vi "ToDegressSetpoint.vi"(4 "Range":cluster{"output high":dbl, "output low":dbl}={"output high"=0.6, "output low"=-0.6} {"output low" format="%.2f"; "output high" format="%.2f"}, 5 "Delay After":i32, 6 "Gains":T1={"proportional gain (Kc)"=1.0, "integral time (Ti, min)"=0.01, "derivative time (Td, min)"=0.0} {"derivative time (Td, min)" format="%.3f"; "integral time (Ti, min)" format="%.3f"; "proportional gain (Kc)" format="%.3f"}, 7 "Loop Wait Delay":i32, 8 "Reset":bool, 9 "Precision":dbl, 10 "Yaw":dbl, 11 "Setpoint (degress)":dbl) -> (0 "Finished?":bool, 3 "Output":dbl)   [LabVIEW 2019]
panel:
  out "PID":cluster{"Distance":dbl, "Encoder Count":dbl}(graph)
  in  "Integral Range":dbl=10000.0
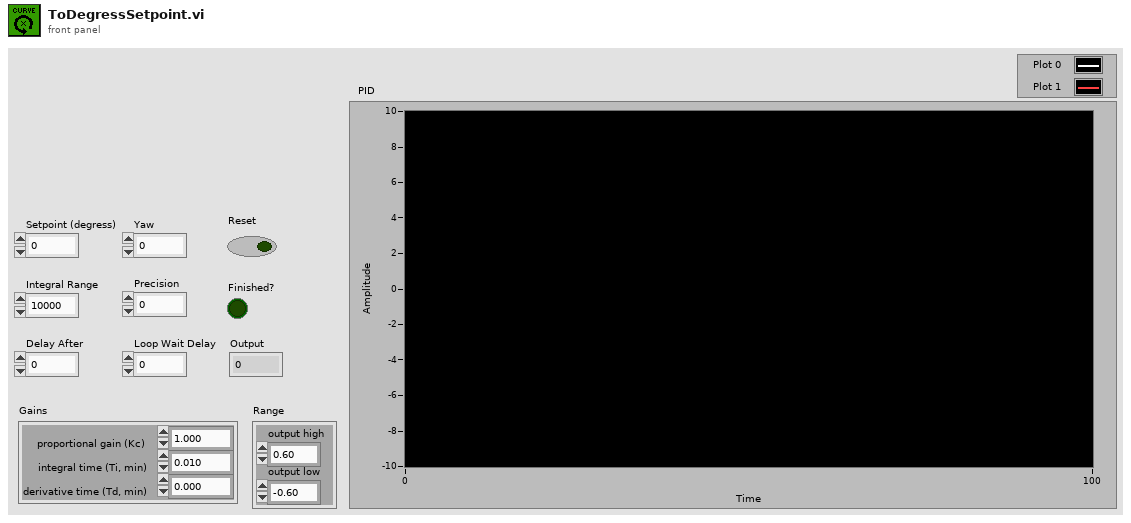
[diagram p1: front panel]
types:
  T1 = cluster{"proportional gain (Kc)":dbl, "integral time (Ti, min)":dbl, "derivative time (Td, min)":dbl}
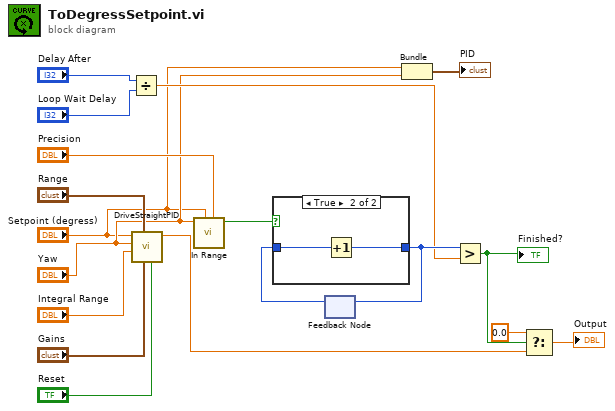
[diagram p0: block diagram]
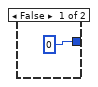
[diagram p2: hidden frame]
diagram:
  n1 = Divide(x="Delay After", y="Loop Wait Delay") -> (x/y=w5:dbl)
  n2 = call "DriveStraightPID.vi"("Reset"="Reset", "Gains"="Gains", "Range"="Range", "Integral Range"="Integral Range", "Process variable"="Yaw", "Setpoint"="Setpoint (degress)") -> ("output"=w8:dbl)  [unwired: 5 in]
  n3 = call "In Range.vi"("Range"="Precision", "Setpoint"="Setpoint (degress)", "Value"="Yaw") -> ("in range?"=w12:bool)  [unwired: 8 in]
  n4 = feedback #1() -> (w10:i32)  [unwired: 1 in]
  n5 = case shown="True" w12 {
    tunnel: [0 w20] -> w6
    tunnel: w10 -> [_ w21]
    frame False {
    }
    frame True {
      n6 = Increment(x=w21) -> (x+1=w20:i32)
    }
  }
  n7 = feedback-in #1(w6) -> ()
  n8 = Bundle("Setpoint (degress)"="Setpoint (degress)", "Yaw"="Yaw") -> (→"PID":cluster{"Setpoint (degress)":dbl, "Yaw":dbl})  [unwired: 1 in]
  n9 = Greater?(x=w6, y=w5) -> (0:w4:bool)
  "Finished?" <- w4
  n10 = Select(t=0.0, s=w4, f=w8) -> (s? t:f=→"Output":dbl)
